vi "loadAmic.vi"(8 "error in":errorcluster, 11 "machine":string) -> (0 "error out":errorcluster)   [LabVIEW 2012]
uses:
  <vilib>/addons/database/Auxilliary.llb/DB Tools Cursor Type.ctl
  <vilib>/addons/database/Connection.llb/DB Tools Open Connec (Path).vi
  <vilib>/addons/database/Connection.llb/Conn Execute.vi
  <vilib>/addons/database/Recordset.llb/Rec Destroy - Connection.vi
  <vilib>/addons/database/NI_Database_API.lvlib
panel:
  out "output cluster":T1
  in  "error in (no error)":errorcluster
  in  "input cluster 2":T1
  out "filenames":string[](array[string])
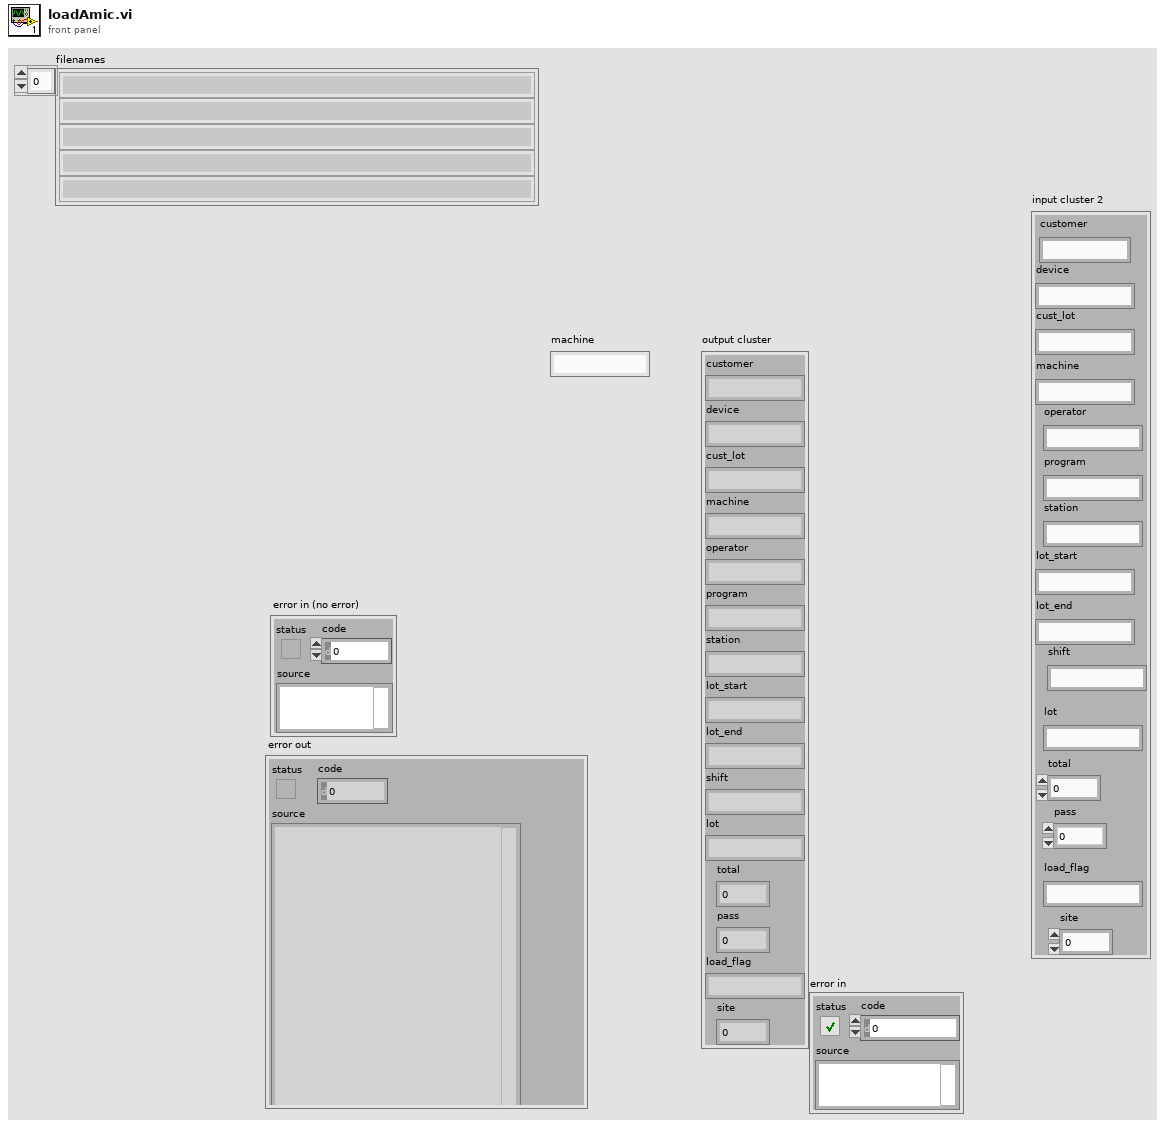
[diagram p1: front panel]
types:
  T1 = cluster{"customer":string, "device":string, "cust_lot":string, "machine":string, "operator":string, "program":string, "station":string, "lot_start":string, "lot_end":string, "shift":string, "lot":string, "total":dbl, "pass":dbl, "load_flag":string, "site":dbl}
  T2 = typedef "NI_Database_API.lvlib/Conn ObjectReference.ctl" = refnum<k1>
  T3 = typedef "NI_Database_API.lvlib/DB Tools Cursor Type.ctl" = enum16{"forward-only", "keyset", "dynamic", "static"}
  T4 = typedef "NI_Database_API.lvlib/Rec ObjectReference.ctl" = refnum<k1>
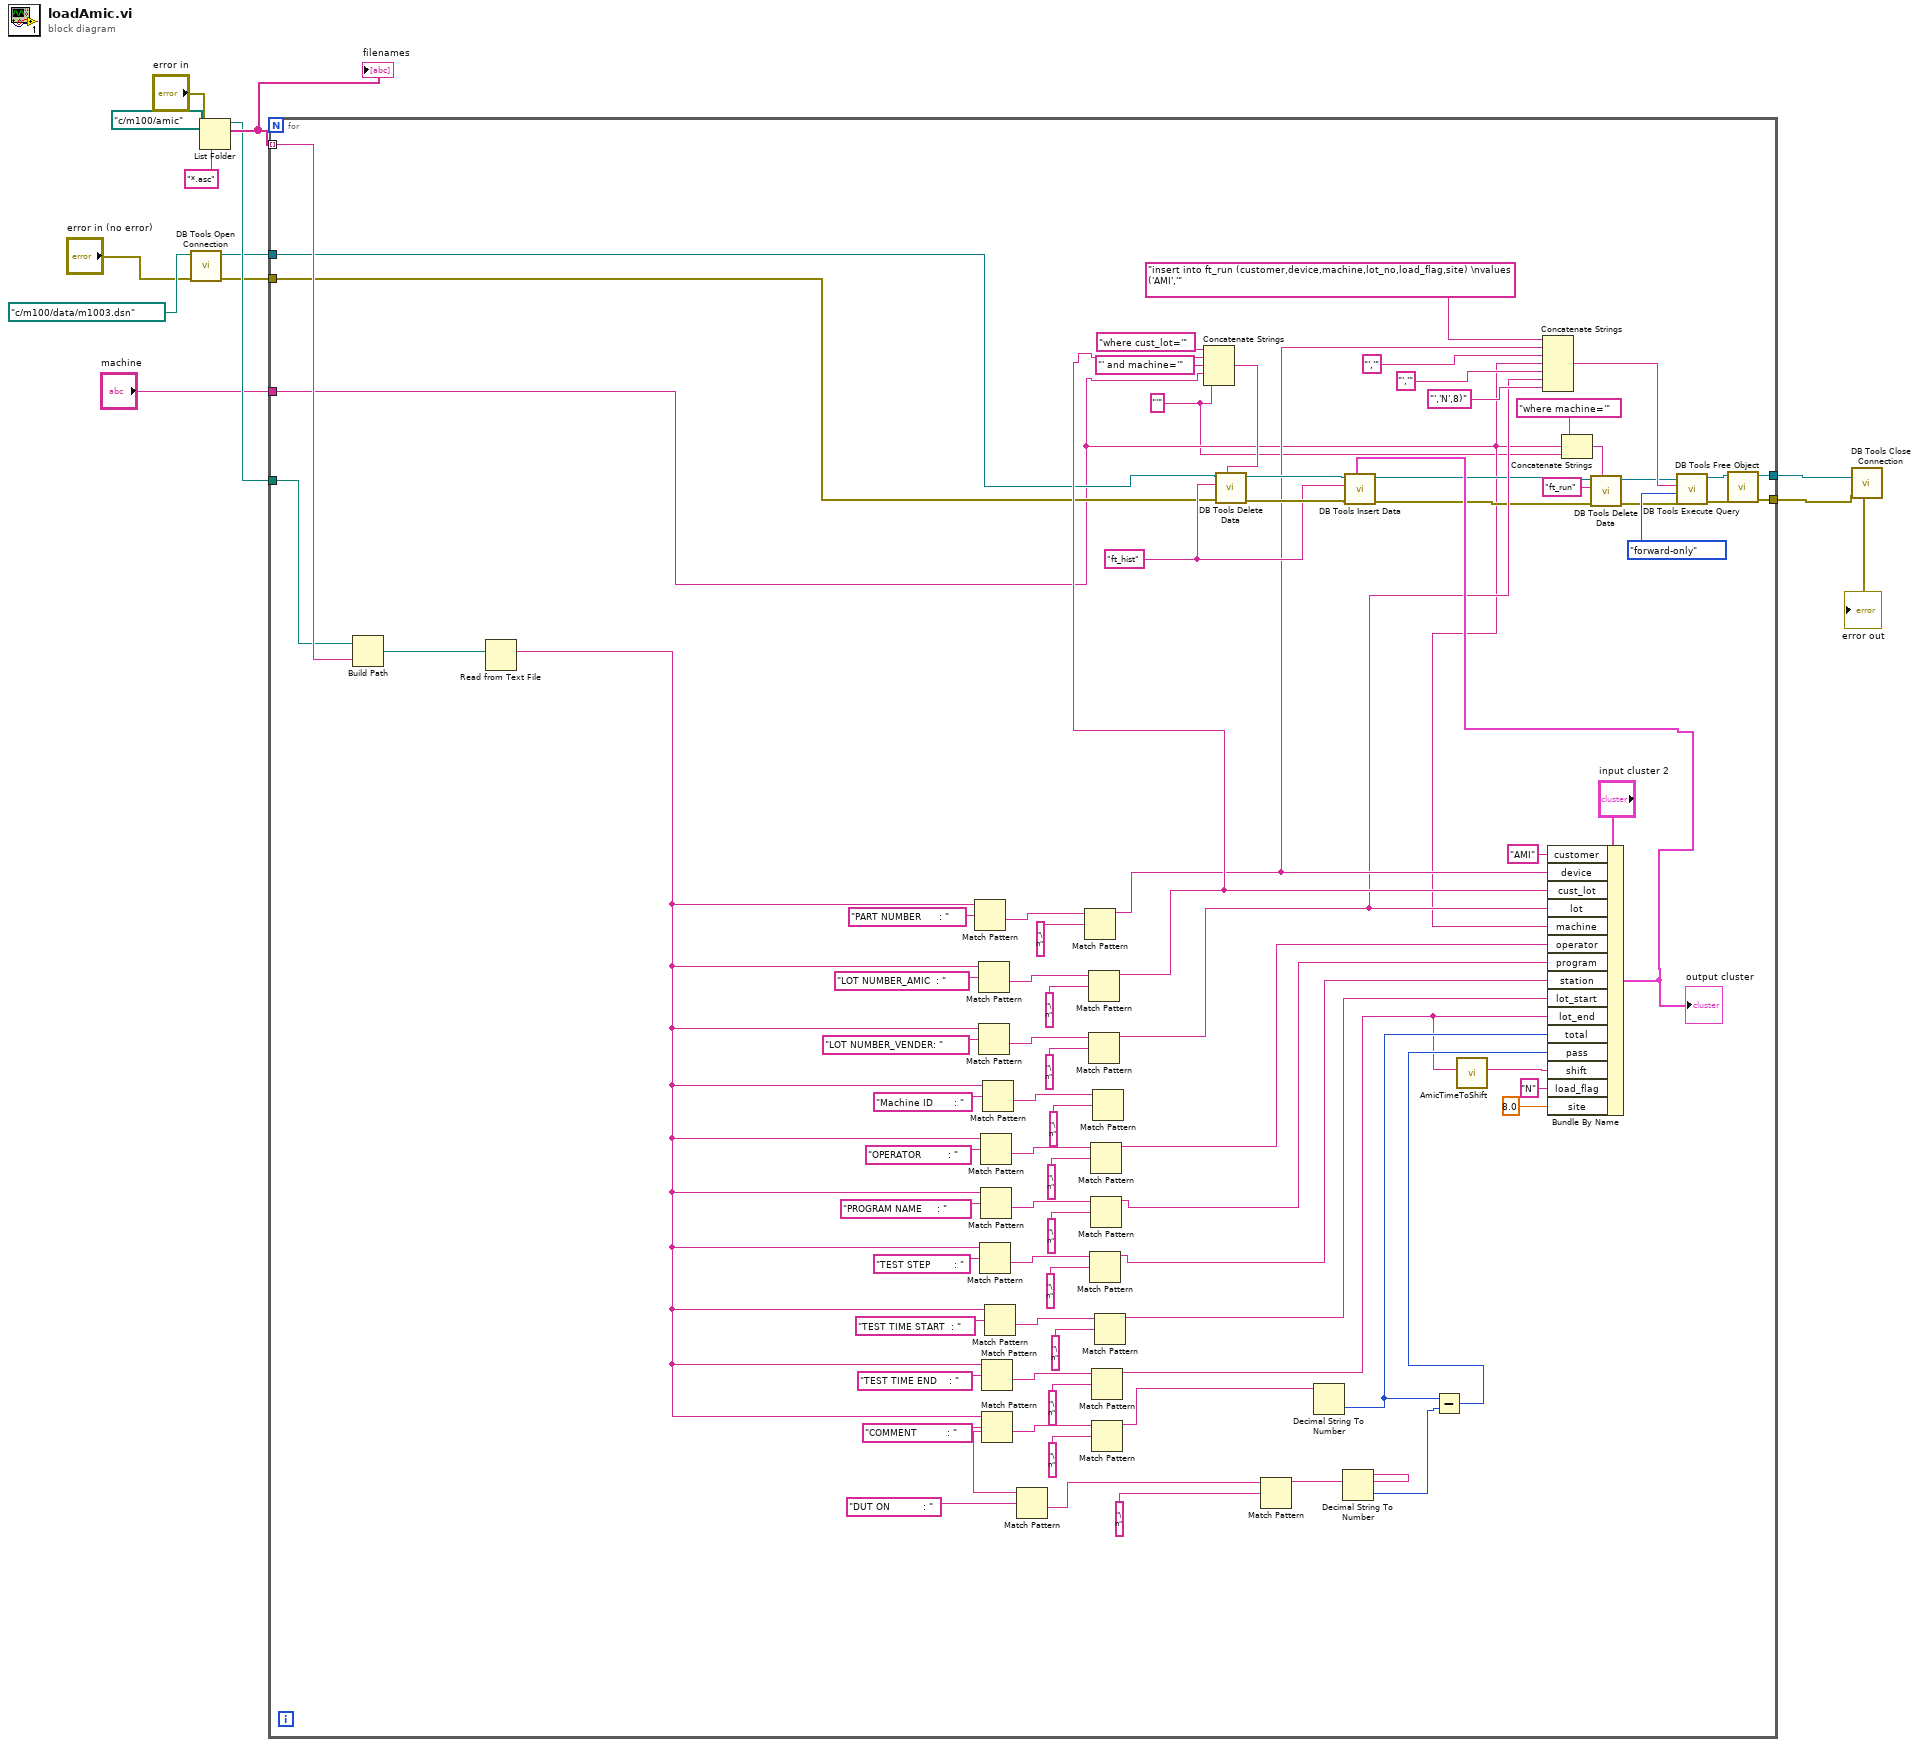
[diagram p0: block diagram]
diagram:
  n1 = call-poly <vilib>:"DB Tools Open Connection.vi"("error in (no error)"="error in (no error)", "connection information"=path "c:/m100/data/m1003.dsn") -> ("error out"=w4:errorcluster, "connection reference"=w5:T2)  [unwired: 6 in]
  n2 = List Folder(path=path "c:/m100/amic", pattern="*.asc", error in="error in") -> (path out=w10:path, filenames=w11:string[])  [unwired: 1 in, 2 out]
  "filenames" <- w11
  n3 = for {
    tunnel: w11 -> [w95] mode=indexing
    tunnel: w10 -> [w94]
    tunnel: "machine" -> [w15]
    tunnel: w5 -> [w31]
    tunnel: w4 -> [w30]
    tunnel: [w26] -> w2
    tunnel: [w25] -> w1
    w14 = "'" ("string")
    w44 = "ft_hist" ("table 2")
    n4 = Build Path(base path=w94, name or relative path=w95) -> (appended path=w96:path)
    n5 = Read from Text File(file (use dialog)=w96) -> (text=w64:string)  [unwired: 3 in, 3 out]
    n6 = Match Pattern(string=w64, regular expression="PART NUMBER      : ") -> (after substring=w92:string)  [unwired: 1 in, 3 out]
    n7 = Match Pattern(string=w64, regular expression="LOT NUMBER_AMIC  : ") -> (after substring=w89:string)  [unwired: 1 in, 3 out]
    n8 = Match Pattern(string=w64, regular expression="LOT NUMBER_VENDER: ") -> (after substring=w86:string)  [unwired: 1 in, 3 out]
    n9 = Match Pattern(string=w64, regular expression="TEST STEP        : ") -> (after substring=w74:string)  [unwired: 1 in, 3 out]
    n10 = Match Pattern(string=w64, regular expression="OPERATOR         : ") -> (after substring=w80:string)  [unwired: 1 in, 3 out]
    n11 = Match Pattern(string=w64, regular expression="PROGRAM NAME     : ") -> (after substring=w77:string)  [unwired: 1 in, 3 out]
    n12 = Match Pattern(string=w64, regular expression="TEST TIME END    : ") -> (after substring=w68:string)  [unwired: 1 in, 3 out]
    n13 = Match Pattern(string=w64, regular expression="COMMENT          : ") -> (after substring=w63:string)  [unwired: 1 in, 3 out]
    n14 = Match Pattern(string=w64, regular expression="Machine ID       : ") -> (after substring=w83:string)  [unwired: 1 in, 3 out]
    n15 = Match Pattern(string=w64, regular expression="TEST TIME START  : ") -> (after substring=w71:string)  [unwired: 1 in, 3 out]
    n16 = Match Pattern(string=w63, regular expression="DUT ON           : ") -> (after substring=w60:string)  [unwired: 1 in, 3 out]
    n17 = Match Pattern(string=w92, regular expression="\n") -> (before substring=w37:string)  [unwired: 1 in, 3 out]
    n18 = Match Pattern(string=w89, regular expression="\n") -> (before substring=w40:string)  [unwired: 1 in, 3 out]
    n19 = Match Pattern(string=w86, regular expression="\n") -> (before substring=w32:string)  [unwired: 1 in, 3 out]
    n20 = Match Pattern(string=w74, regular expression="\n") -> (before substring=w54:string)  [unwired: 1 in, 3 out]
    n21 = Match Pattern(string=w80, regular expression="\n") -> (before substring=w56:string)  [unwired: 1 in, 3 out]
    n22 = Match Pattern(string=w77, regular expression="\n") -> (before substring=w55:string)  [unwired: 1 in, 3 out]
    n23 = Match Pattern(string=w68, regular expression="\n") -> (before substring=w34:string)  [unwired: 1 in, 3 out]
    n24 = Match Pattern(string=w63, regular expression="\n") -> (before substring=w59:string)  [unwired: 1 in, 3 out]
    n25 = Match Pattern(string=w83, regular expression="\n") -> ()  [unwired: 1 in, 4 out]
    n26 = Match Pattern(string=w71, regular expression="\n") -> (before substring=w53:string)  [unwired: 1 in, 3 out]
    n27 = Concatenate Strings("where cust_lot='" ("string"), w40, "' and machine='" ("string"), w15, w14) -> (w18:string)
    n28 = call <vilib>:"DB Tools Delete Data.vi"("condition"=w18, "error in (no error)"=w30, "table"=w44, "connection reference"=w31) -> ("error out"=w45:errorcluster, "connection reference out"=w46:T2)  [unwired: 6 in]
    n29 = Match Pattern(string=w60, regular expression="\n") -> (before substring=w58:string)  [unwired: 1 in, 3 out]
    n30 = Decimal String To Number(string=w59) -> (number=w48:i32)  [unwired: 2 in, 1 out]
    n31 = Decimal String To Number(string=w58) -> (number=w49:i32)  [unwired: 2 in, 1 out]
    n32 = Subtract(x=w48, y=w49) -> (x-y=w47:i32)
    n33 = call "AmicTimeToShift.vi"("input string"=w34) -> ("s? t:f"=w50:string)  [unwired: 10 in]
    n34 = Concatenate Strings("insert into ft_run (customer,device,machine,lot_no,load_flag,site) \nvalues ('AMI','" ("string"), w37, "','" ("string"), w15, "','" ("string"), w32, "','N',8)" ("string")) -> (w24:string)
    n35 = Bundle By Name(cluster="input cluster 2", "customer"="AMI", "device"=w37, "cust_lot"=w40, "lot"=w32, "machine"=w15, "operator"=w56, "program"=w55, "station"=w54, "lot_start"=w53, "lot_end"=w34, "total"=w48, "pass"=w47, "shift"=w50, "load_flag"="N", "site"=8.0) -> (w41:T1)
    "output cluster" <- w41
    n36 = call <vilib>:"DB Tools Insert Data.vi"("data"=w41, "error in (no error)"=w45, "table"=w44, "connection reference"=w46) -> ("error out"=w22:errorcluster, "connection reference out"=w23:T2)  [unwired: 6 in]
    n37 = Concatenate Strings("where machine='" ("string"), w15, w14) -> (w17:string)
    n38 = call <vilib>:"DB Tools Delete Data.vi"("condition"=w17, "error in (no error)"=w22, "table"="ft_run", "connection reference"=w23) -> ("error out"=w20:errorcluster, "connection reference out"=w21:T2)  [unwired: 6 in]
    n39 = call-poly <vilib>:"DB Tools Execute Query.vi"("error in (no error)"=w20, "cursor type"=DB_Tools_Cursor_Type."forward-only", "SQL query"=w24, "connection reference"=w21) -> ("error out"=w28:errorcluster, "recordset reference"=w27:T4)  [unwired: 4 in]
    n40 = call-poly <vilib>:"DB Tools Free Object.vi"("error in (no error)"=w28, "recordset reference"=w27) -> ("error out"=w25:errorcluster, "connection reference"=w26:T2)  [unwired: 8 in]
  }
  n41 = call <vilib>:"DB Tools Close Connection.vi"("error in (no error)"=w1, "connection reference"=w2) -> ("error out"=→"error out":errorcluster)  [unwired: 5 in]
